vi "MCB2300 AI Specify Node.vi"(10 "Node Attributes":T1) -> (3 "type out":T2)   [LabVIEW 2011]
doc: "This VI is a \"Specify Node\" vi. It is used to pick which I/O Implementation VI to use when more than one is specified for an I/O resource. This VI looks at the Node Attributes and selects the type of the I/O based on whether the user selects array or scalar data and whether they select scaled or raw binary. The output is a variant that indicates the type returned by the I/O and it must match the type of one of the I/O Implementation VIs."
uses:
  <vilib>/eio/EIO_TypeDescriptor.ctl
  <vilib>/Embedded/ARM/MCB2300/MCB2300_AI_NodeAttr.ctl
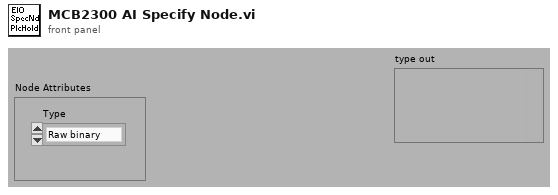
[diagram p1: front panel]
types:
  T1 = typedef "MCB2300_AI_NodeAttr.ctl" = cluster{"Type":enum16{"Raw binary", "Scaled voltage"}}
  T2 = typedef "EIO_TypeDescriptor.ctl" = variant
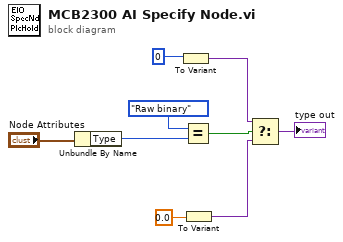
[diagram p0: block diagram]
diagram:
  n1 = Unbundle By Name("Node Attributes") -> ("Type"=w4:enum16{"Raw binary", "Scaled voltage"})
  n2 = To Variant(anything=u32 0) -> (Variant=w7:variant)
  n3 = Equal?(x=enum16{"Raw binary", "Scaled voltage"}."Raw binary" ("Type"), y=w4) -> (x = y?=w3:bool)
  n4 = To Variant(anything=0.0) -> (Variant=w8:variant)
  n5 = Select(t=w7, s=w3, f=w8) -> (s? t:f=→"type out":variant)
